vi "SetData.vi"(6 "PayloadType":u16, 8 "error in (no error)":errorcluster, 9 "Payload":string, 10 "NodeID":string, 11 "DataPacket in":refnum<class "DataPacket.lvclass">) -> (0 "error out":errorcluster, 3 "DataPacket out":refnum<class "DataPacket.lvclass">)   [LabVIEW 2021, in "DataPacket.lvclass"]
uses:
  DataPacket.lvclass
  DataPacket.lvclass/DataPacket.ctl
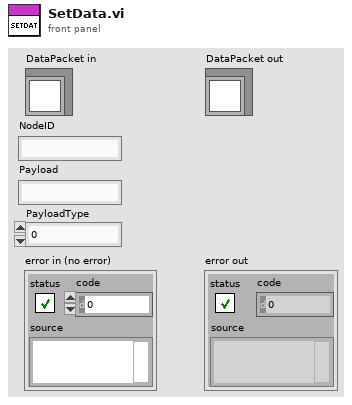
[diagram p1: front panel]
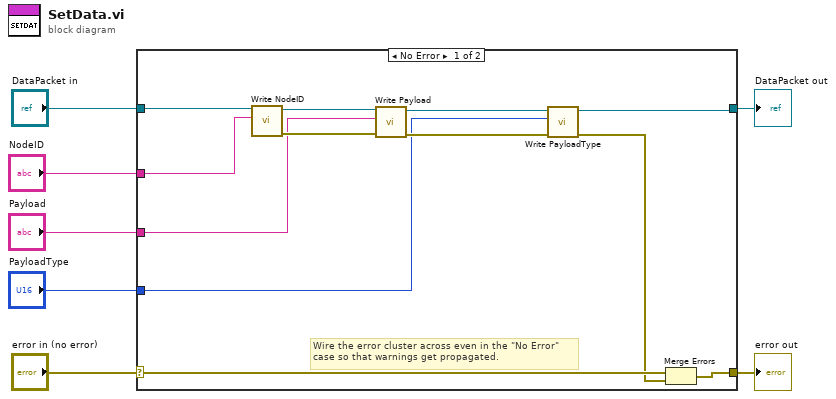
[diagram p0: block diagram]
diagram:
  n1 = case shown="No Error" "error in (no error)" {
    selector: "error in (no error)" -> [w19 w21]
    tunnel: [w12 w21] -> w6
    tunnel: [w13 w20] -> w4
    tunnel: "DataPacket in" -> [w14 w20]
    tunnel: "NodeID" -> [w10 _]
    tunnel: "Payload" -> [w9 _]
    tunnel: "PayloadType" -> [w8 _]
    frame No Error {
      # "Wire the error cluster across even in the \"No Error\"\ncase so that warnings get propagated."
      n2 = call "Write NodeID.vi"("NodeID"=w10, "DataPacket in"=w14) -> ("error out"=w17:errorcluster, "DataPacket out"=w18:refnum<class "DataPacket.lvclass">)  [unwired: 8 in]
      n3 = call "Write Payload .vi"("error in (no error)"=w17, "Payload"=w9, "DataPacket in"=w18) -> ("error out"=w15:errorcluster, "DataPacket out"=w16:refnum<class "DataPacket.lvclass">)  [unwired: 7 in]
      n4 = call "Write PayloadType.vi"("error in (no error)"=w15, "PayloadType"=w8, "DataPacket in"=w16) -> ("error out"=w11:errorcluster, "DataPacket out"=w13:refnum<class "DataPacket.lvclass">)  [unwired: 7 in]
      n5 = Merge Errors(w19, w11) -> (w12:errorcluster)
    }
    frame Error {
    }
  }
  "error out" <- w6
  "DataPacket out" <- w4
